vi "Data Source 2 LBCB Number.vi"(10 "Dataset Source":T2) -> (2 "LBCB Number":T1)   [LabVIEW 2013]
uses:
  Dataset Source.ctl
  Data Access Objects/Metadata/LBCB Number.ctl
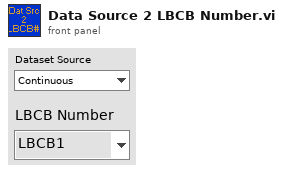
[diagram p1: front panel]
types:
  T1 = typedef "LBCB Number.ctl" = enum16{"LBCB1", "LBCB2"}
  T2 = typedef "Dataset Source.ctl" = enum16{"Continuous", "Hold", "ED", "Volts", "Offsets", "Increments"}
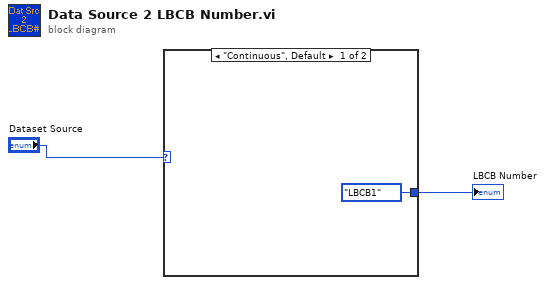
[diagram p0: block diagram]
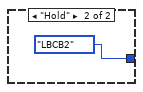
[diagram p2: hidden frame]
diagram:
  n1 = case shown="\"Continuous\", Default" "Dataset Source" {
    tunnel: [LBCB_Number."LBCB1" ("LBCB Number") LBCB_Number."LBCB2" ("LBCB Number")] -> w1
    frame "Continuous", Default {
    }
    frame "Hold" {
    }
  }
  "LBCB Number" <- w1
